vi "close.vi"(8 "error in (no error)":errorcluster, 11 "ScintillaNET in":refnum<class "ScintillaNET.lvclass">) -> (0 "error out":errorcluster)   [LabVIEW 2018, in "ScintillaNET.lvclass"]
uses:
  ScintillaNET.lvclass
  ScintillaNET.lvclass/ScintillaNET.ctl
  D:/project/hobby/LabVIEW/LF2R/LabVIEW/Source/ScintillaNET/dll/ScintillaNET.dll
  dll/ScintillaNET.dll
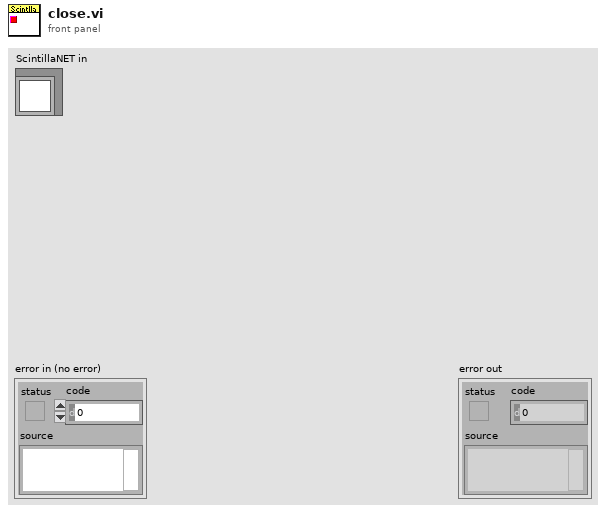
[diagram p1: front panel]
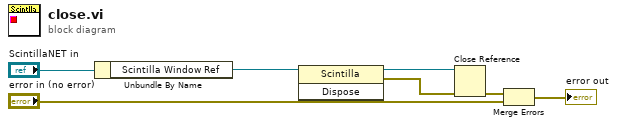
[diagram p0: block diagram]
diagram:
  n1 = Unbundle By Name("ScintillaNET in") -> ("Scintilla Window Ref"=w1:refnum<k24>)
  n2 = invoke class="Scintilla" method="Dispose"(reference=w1) -> (reference out=w3:refnum<k24>, error out=w2:errorcluster)  [unwired: 2 in, 1 out]
  n3 = Close Reference(reference=w3, error in (no error)=w2) -> (error out=w6:errorcluster)
  n4 = Merge Errors(w6, "error in (no error)") -> (→"error out":errorcluster)
